vi "test.vi"() -> ()   [LabVIEW 2019]
uses:
  c83abc26-5a52-4cfa-9df0-9e96a6eb4de7.vi
  7465a6ab-5d66-4325-99fb-652503195ccb.vi
panel:
  out "output 2":dbl
  out "output 1":string
  in  "Command":string
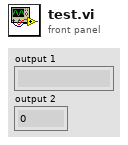
[diagram p1: front panel]
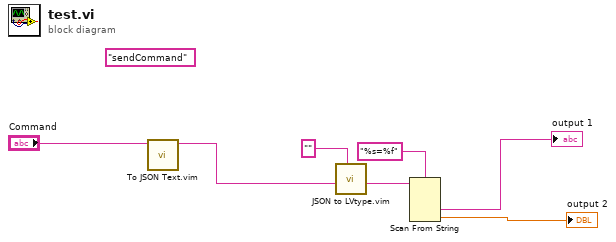
[diagram p0: block diagram]
diagram:
  (unwired) "sendCommand" ("Message.Command")
  n1 = call "To JSON Text.vim"("Anything"="Command") -> ("<JSON>"=w3:string)  [unwired: 9 in, 1 out]
  n2 = call "JSON to LVtype.vim"("type"="", "JSON Data in"=w3) -> ("Data out"=w5:string)  [unwired: 8 in, 1 out]
  n3 = Scan From String(format string="%s=%f", input string=w5) -> (output 1=→"output 1":string, output 2=→"output 2":dbl)  [unwired: 4 in, 3 out]
